vi "CreateProjectsForEachLibrary.vi"() -> ()   [LabVIEW 2023, in "DepsWatchToolsMenu.lvlib"]
uses:
  DepsWatchToolsMenu.lvlib
  <userlib>/_OpenG.lib/file/file.llb/Append Path to Root if Relative - Scalar__ogtk.vi
  <userlib>/_OpenG.lib/file/file.llb/Compare Two Paths - Scalar__ogtk.vi
  <userlib>/_OpenG.lib/file/file.llb/openg_file.lvlib
  vi.lib/DepsWatch/DepsWatch.lvlib
panel:
  out "Projects Created":path[](array[path])
  out "error out":errorcluster
  in  "Build Specs Folder Path":path=path "C:/sw-deps-monitor/Source/BuildSpecs"
  in  "error in (no error)":errorcluster
  in  "Source Folder Path":path=path "C:/sw-deps-monitor/Source"
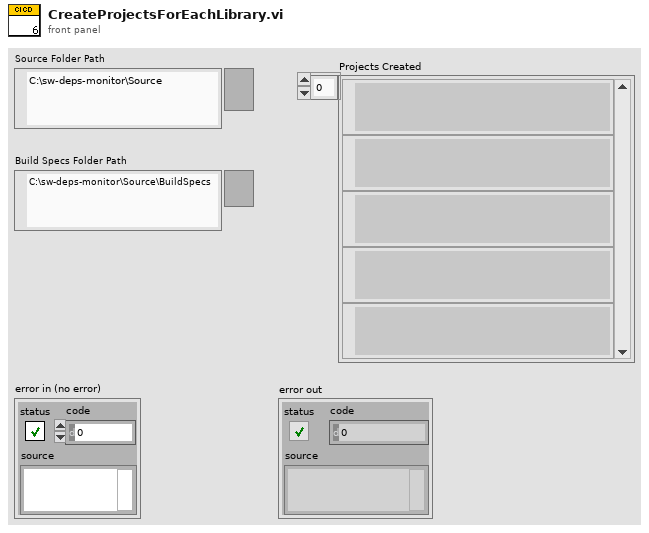
[diagram p1: front panel]
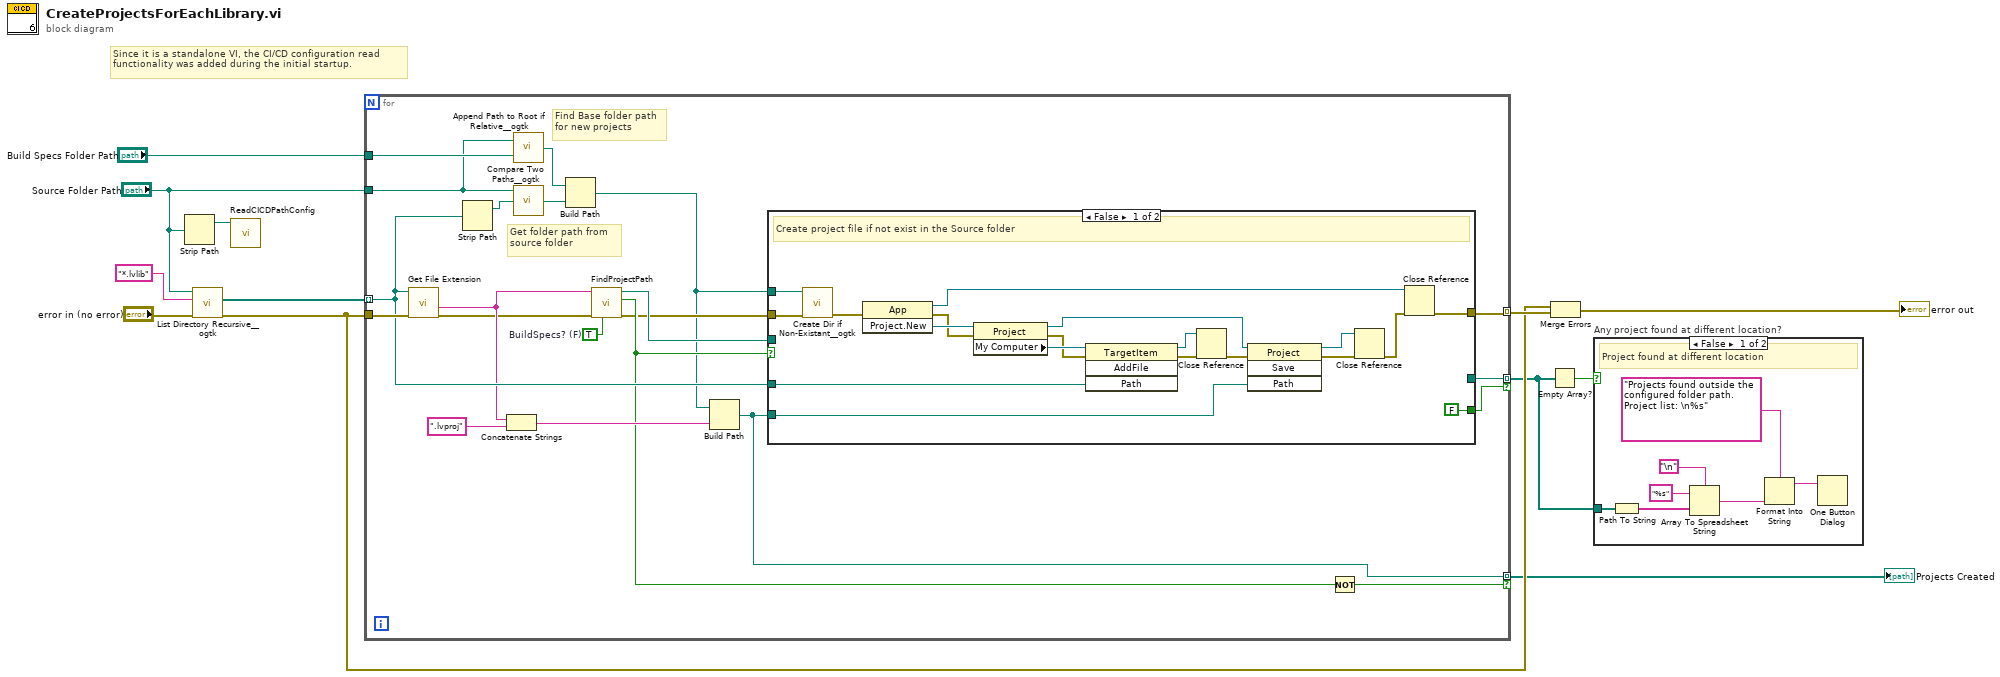
[diagram p0: block diagram]
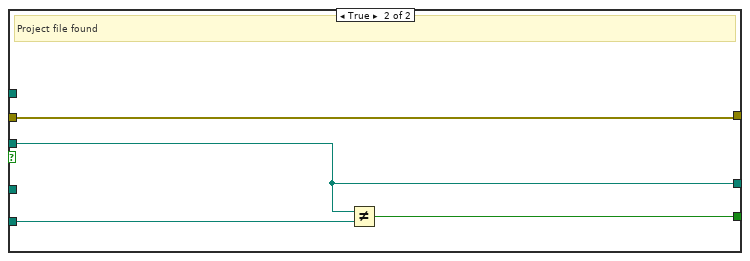
[diagram p3: hidden frame]
diagram:
  # "Since it is a standalone VI, the CI/CD configuration read functionality was added during the initial startup."
  n1 = Strip Path(path="Source Folder Path") -> (stripped path=w1:path)  [unwired: 1 out]
  n2 = call <userlib>:"List Directory Recursive__ogtk.vi"("error in (no error)"="error in (no error)", "pattern"="*.lvlib", "Path"="Source Folder Path") -> ("error out"=w7:errorcluster, "file paths"=w10:path[])  [unwired: 5 in, 2 out]
  n3 = call "ReadCICDPathConfig.vi"("Workspace Path"=w1) -> ()  [unwired: 9 in, 2 out]
  n4 = for {
    tunnel: w7 -> [w33]
    tunnel: w10 -> [w29] mode=indexing
    tunnel: "Build Specs Folder Path" -> [w26]
    tunnel: [w30] -> w8 mode=indexing
    tunnel: [w28] -> w5 mode=indexing if=w27
    tunnel: "Source Folder Path" -> [w25]
    tunnel: [w16] -> w3 mode=indexing if=w15
    w22 = TRUE  # BuildSpecs? (F)
    # "Find Base folder path for new projects"
    # "Get folder path from source folder"
    n5 = call <vilib>:"Get File Extension.vi"("error in (no error)"=w33, "file"=w29) -> ("error out"=w23:errorcluster, "filename without extension"=w24:string)  [unwired: 5 in, 3 out]
    n6 = Strip Path(path=w29) -> (stripped path=w21:path)  [unwired: 1 out]
    n7 = Concatenate Strings(w24, ".lvproj" ("string")) -> (w31:string)
    n8 = call-poly <userlib>:"Append Path to Root if Relative__ogtk.vi"("Absolute or Relative Path"=w26, "Root Path"=w25) -> ("Absolute or Appended Path"=w20:path)
    n9 = call-poly <userlib>:"Compare Two Paths__ogtk.vi"("path2"=w21, "path1"=w25) -> ("relative path from 1 to 2"=w19:path)  [unwired: 1 in, 2 out]
    n10 = Build Path(base path=w20, name or relative path=w19) -> (appended path=w13:path)
    n11 = call "FindProjectPath.vi"("BuildSpecs? (F)"=w22, "error in (no error)"=w23, "Library Name"=w24) -> ("error out"=w14:errorcluster, "Found?"=w18:bool, "Project Path"=w17:path)  [unwired: 6 in]
    n12 = Build Path(base path=w13, name or relative path=w31) -> (appended path=w28:path)
    n13 = case shown="False" w18 {
      tunnel: [w52 w56] -> w30
      tunnel: w29 -> [w51 _]
      tunnel: w14 -> [w36 w56]
      tunnel: w28 -> [w38 w55]
      tunnel: w17 -> [_ w54]
      tunnel: [_ w54] -> w16
      tunnel: [FALSE w53] -> w15
      tunnel: w13 -> [w35 _]
      frame False {
        # "Create project file if not exist in the Source folder"
        n14 = call <userlib>:"Create Dir if Non-Existant__ogtk.vi"("error in (no error)"=w36, "Directory Path"=w35) -> ("error out"=w34:errorcluster)  [unwired: 7 in, 2 out]
        n15 = invoke class="App" method="Project.New"(error in=w34) -> (reference out=w49:refnum<vi>, error out=w48:errorcluster, "Project:New"=w50:refnum<vi>)  [unwired: 2 in]
        n16 = property class="Project"(reference=w50, error in=w48) -> (reference out=w41:refnum<vi>, error out=w46:errorcluster, "My Computer"=w47:refnum<vi>)
        n17 = invoke class="TargetItem" method="AddFile"(reference=w47, error in=w46, "Path"=w51) -> (reference out=w45:refnum<vi>, error out=w44:errorcluster)  [unwired: 1 in, 2 out]
        n18 = Close Reference(reference=w45, error in (no error)=w44) -> (error out=w42:errorcluster)
        n19 = invoke class="Project" method="Save"(reference=w41, error in=w42, "Path"=w38) -> (reference out=w40:refnum<vi>, error out=w39:errorcluster)  [unwired: 1 in, 2 out]
        n20 = Close Reference(reference=w40, error in (no error)=w39) -> (error out=w43:errorcluster)
        n21 = Close Reference(reference=w49, error in (no error)=w43) -> (error out=w52:errorcluster)
      }
      frame True {
        # "Project file found"
        n22 = Not Equal?(x=w54, y=w55) -> (x != y?=w53:bool)
      }
    }
    n23 = Not(x=w18) -> (.not. x?=w27:bool)
  }
  "Projects Created" <- w5
  n24 = Empty Array?(array=w3) -> (empty?=w4:bool)
  n25 = Merge Errors(w7, w8) -> (→"error out":errorcluster)
  n26 = case "Any project found at different location?" shown="False" w4 {
    tunnel: w3 -> [w63 _]
    frame False {
      # "Project found at different location"
      n27 = Path To String(path=w63) -> (string=w60:string[])
      n28 = Array To Spreadsheet String(delimiter (Tab)="\n", array=w60, 3:"%s" ("format string")) -> (spreadsheet string=w59:string)
      n29 = Format Into String(format string="Projects found outside the configured folder path. Project list: \n%s", w59) -> (resulting string=w58:string)  [unwired: 2 in, 1 out]
      n30 = One Button Dialog(message=w58) -> ()  [unwired: 1 in, 1 out]
    }
    frame True {
    }
  }
